vi "Lin_Rohner_lab4A_Stiction torque.vi"() -> ()   [LabVIEW 2019]
uses:
  <vilib>/Analysis/3filter.llb/Filter Passband Type.ctl
  <vilib>/Platform/TimedLoop/XDataNode/timing_clust.ctl
  <vilib>/Platform/TimedLoop/XDataNode/nitl_modes.ctl
  <vilib>/Platform/TimedLoop/XDataNode/wakeup.ctl
  <vilib>/DAQmx/write.llb/DAQmx Write (Analog DBL 1Chan 1Samp).vi
  <vilib>/DAQmx/read.llb/DAQmx Read (Analog DBL 1Chan 1Samp).vi
  <vilib>/DAQmx/create/channels.llb/DAQmx Create Channel (AO-Voltage-Basic).vi
  <vilib>/DAQmx/miscellaneous.llb/DAQmx Fill In Error Info.vi
  <vilib>/DAQmx/create/channels.llb/DAQmx Create Channel (AI-Voltage-Basic).vi
  <vilib>/platform/TimedLoop/XDataNode/XDataNode.xnode
  <vilib>/Platform/TimedLoop/XDataNode/XDNodeRunTimeDep.lvlib
  <vilib>/ptbypt/NI_PtbyPt.lvlib
  <vilib>/Analysis/NI_AALBase.lvlib
panel:
  out "Start Position":dbl
  out "Delta Position":dbl
  in  "Go!":bool
  out "Filtered Position":dbl(graph)
  out "Filtered Position":dbl
  in  "low cutoff freq: Position":dbl=0.125 format="%0.3f"
  out "Motor Voltage":dbl
  out "Motor Current":dbl(graph)
  out "Motor Current":dbl
  out "Motor Control Voltage":dbl(graph)
  in  "Stop!":bool
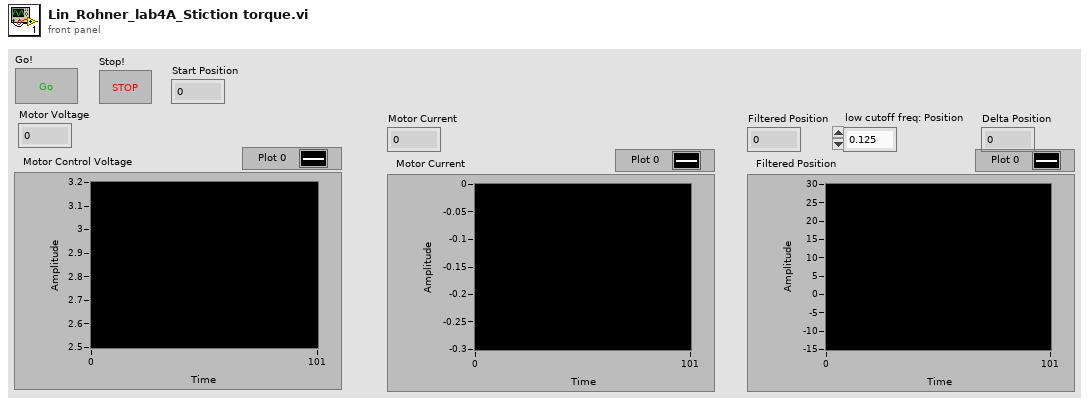
[diagram p1: front panel]
types:
  T1 = typedef "NI_AALBase.lvlib/Filter Passband Type.ctl" = enum32{"Lowpass", "Highpass", "Bandpass", "Bandstop"}
  T2 = typedef "XDNodeRunTimeDep.lvlib/timing_clust.ctl" = cluster{"Expected End [f-1]":u64, "Actual End [f-1]":u64, "Finished Late? [f-1]":bool, "Expected End [i-1]":u64, "Actual End [i-1]":u64, "Finished Late? [i-1]":bool, "Expected Start [i]":u64, "Actual Start [i]":u64, "Expected Start [f]":u64, "Actual Start [f]":u64, "Source Name":string, "Structure Name":string, "Period":i64, "Deadline":i64, "Offset":i64, "Start":i64, "Priority":i32, "Timeout":i32, "Mode":T3, "Wakeup Reason":T4, "Error":errorcluster, "Source Type":string, "Secondary Source Type":string, "Global End Time":u64, "Global Start Time":u64, "Frame Duration":u64, "Iteration Duration":u64, "Assigned CPU":i32, "I/O Scan Engine Mode":u32}
  T3 = typedef "XDNodeRunTimeDep.lvlib/nitl_modes.ctl" = enum32{"No Change", "Process missed periods, maintain original phase", "Discard missed periods, maintain original phase", "Process missed periods, ignore original phase", "Discard missed periods, ignore original phase"}
  T4 = typedef "XDNodeRunTimeDep.lvlib/wakeup.ctl" = enum32{"Normal", "Aborted", "Asynchronous wakeup", "Timing source error", "Timed loop error", "Timeout"}
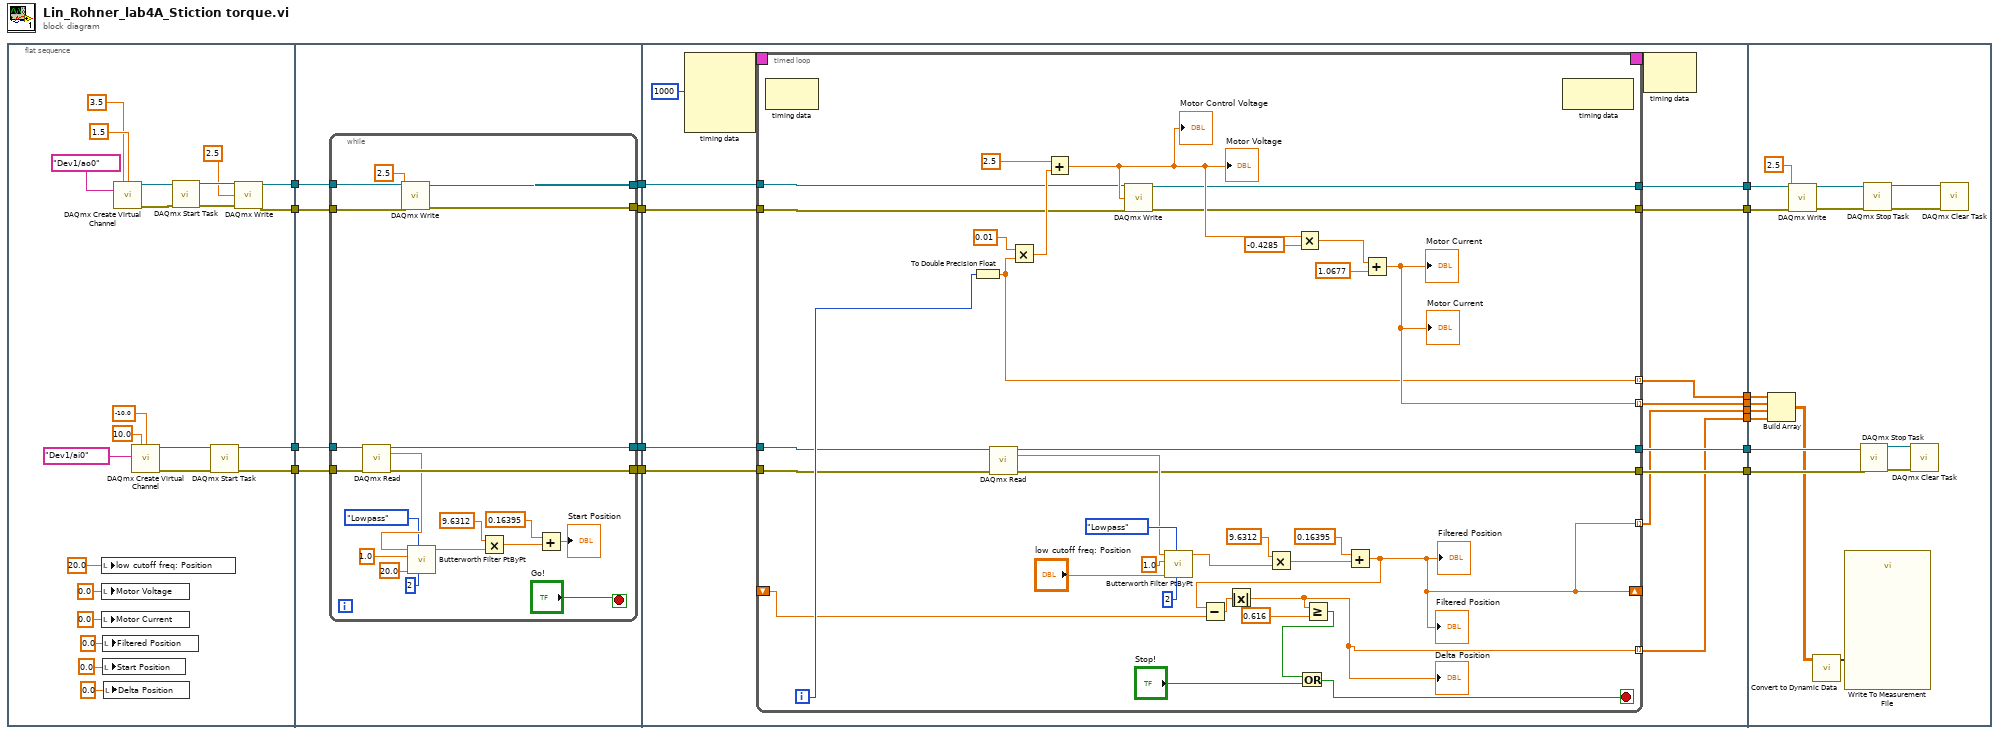
[diagram p0: block diagram]
diagram:
  n1 = flat-sequence {
    tunnel: [w37] -> w11
    tunnel: [w36] -> w9
    tunnel: [w24] -> w7
    tunnel: [w23] -> w5
    tunnel: w11 -> [w47]
    tunnel: [w45] -> w10
    tunnel: w9 -> [w46]
    tunnel: [w44] -> w8
    tunnel: w7 -> [w43]
    tunnel: [w40] -> w6
    tunnel: w5 -> [w42]
    tunnel: [w41] -> w4
    tunnel: w10 -> [w79]
    tunnel: w8 -> [w78]
    tunnel: w6 -> [w77]
    tunnel: w4 -> [w76]
    tunnel: [w75] -> w16
    tunnel: [w74] -> w15
    tunnel: [w73] -> w14
    tunnel: [w72] -> w13
    tunnel: [w71] -> w12
    tunnel: [w70] -> w3
    tunnel: [w69] -> w2
    tunnel: [w68] -> w1
    tunnel: w16 -> [w133]
    tunnel: w15 -> [w132]
    tunnel: w14 -> [w131]
    tunnel: w13 -> [w130]
    tunnel: w12 -> [w128]
    tunnel: w3 -> [w129]
    tunnel: w2 -> [w124]
    tunnel: w1 -> [w125]
    frame #0 {
      n2 = local write "low cutoff freq: Position"(20.0 ("low cutoff freq: Position")) -> ()
      n3 = local write "Motor Voltage"(0.0 ("Motor Voltage")) -> ()
      n4 = local write "Motor Current"(0.0 ("Motor Current")) -> ()
      n5 = local write "Filtered Position"(0.0 ("Filtered Position")) -> ()
      n6 = local write "Start Position"(0.0 ("Start Position")) -> ()
      n7 = local write "Delta Position"(0.0 ("Delta Position")) -> ()
      n8 = call-poly <vilib>:"DAQmx Create Virtual Channel.vi"("maximum value"=3.5, "minimum value"=1.5, "physical channels"=tag "Dev1/ao0") -> ("task out"=w39:refnum<k21>, "error out"=w35:errorcluster)  [unwired: 11 in]
      n9 = call-poly <vilib>:"DAQmx Create Virtual Channel.vi"("maximum value"=10.0, "minimum value"=-10.0, "physical channels"=tag "Dev1/ai0") -> ("task out"=w25:refnum<k21>, "error out"=w26:errorcluster)  [unwired: 11 in]
      n10 = call <vilib>:"DAQmx Start Task.vi"("task/channels in"=w39, "error in"=w35) -> ("task out"=w38:refnum<k21>, "error out"=w34:errorcluster)  [unwired: 12 in]
      n11 = call <vilib>:"DAQmx Start Task.vi"("task/channels in"=w25, "error in"=w26) -> ("task out"=w24:refnum<k21>, "error out"=w23:errorcluster)  [unwired: 12 in]
      n12 = call-poly <vilib>:"DAQmx Write.vi"("task/channels in"=w38, "data"=2.5, "error in"=w34) -> ("task out"=w37:refnum<k21>, "error out"=w36:errorcluster)  [unwired: 10 in, 1 out]
    }
    frame #1 {
      n13 = while {
        tunnel: w47 -> [w67]
        tunnel: w46 -> [w65]
        tunnel: [w66] -> w45
        tunnel: [w64] -> w44
        tunnel: w43 -> [w61]
        tunnel: w42 -> [w58]
        tunnel: [w59] -> w41
        tunnel: [w60] -> w40
        stop <- "Go!" stop-if-true
        n14 = call-poly <vilib>:"DAQmx Read.vi"("task/channels in"=w61, "error in"=w58) -> ("task out"=w60:refnum<k21>, "data"=w57:dbl, "error out"=w59:errorcluster)  [unwired: 11 in]
        n15 = call-poly <vilib>:"DAQmx Write.vi"("task/channels in"=w67, "data"=2.5, "error in"=w65) -> ("task out"=w66:refnum<k21>, "error out"=w64:errorcluster)  [unwired: 10 in, 1 out]
        n16 = call <vilib>:"Butterworth Filter PtByPt.vi"("order"=2, "filter type"=Filter_Passband_Type."Lowpass", "low cutoff freq: fl"=20.0, "sampling freq: fs"=1.0, "x"=w57) -> ("Filtered x"=w49:dbl)  [unwired: 4 in, 1 out]
        n17 = Multiply(x=9.6312, y=w49) -> (x*y=w51:dbl)
        n18 = Add(x=0.16395, y=w51) -> (x+y=→"Start Position":dbl)
      }
    }
    frame #2 {
      n19 = node-c288(i64 1000 ("Period")) -> (w82:T2)  [unwired: 3 in]
      n20 = timed-loop {
        timing: w82 -> [_]
        timing-out: [_] -> w81
        tunnel: w79 -> [w101]
        tunnel: w78 -> [w100]
        tunnel: w77 -> [w97]
        tunnel: w76 -> [w96]
        tunnel: [w99] -> w75
        tunnel: [w98] -> w74
        tunnel: [w95] -> w73
        tunnel: [w94] -> w72
        tunnel: [w89] -> w71 mode=indexing
        shift-right: [w83] -> _
        shift-left: _ -> [w87]
        tunnel: [w85] -> w70 mode=indexing
        tunnel: [w84] -> w69 mode=indexing
        tunnel: [w83] -> w68 mode=indexing
        i -> [w102]
        stop <- w90 stop-if-true
        n21 = node-c288() -> ()  [unwired: 1 in, 1 out]
        n22 = To Double Precision Float(number=w102) -> (double precision float=w85:dbl)
        n23 = call-poly <vilib>:"DAQmx Read.vi"("task/channels in"=w97, "error in"=w96) -> ("task out"=w95:refnum<k21>, "data"=w103:dbl, "error out"=w94:errorcluster)  [unwired: 11 in]
        n24 = Multiply(x=0.01, y=w85) -> (x*y=w116:dbl)
        n25 = Add(x=2.5, y=w116) -> (x+y=w111:dbl)
        "Motor Control Voltage" <- w111
        "Motor Voltage" <- w111
        n26 = call-poly <vilib>:"DAQmx Write.vi"("task/channels in"=w101, "data"=w111, "error in"=w100) -> ("task out"=w99:refnum<k21>, "error out"=w98:errorcluster)  [unwired: 10 in, 1 out]
        n27 = call <vilib>:"Butterworth Filter PtByPt.vi"("order"=2, "filter type"=Filter_Passband_Type."Lowpass", "low cutoff freq: fl"="low cutoff freq: Position", "sampling freq: fs"=1.0, "x"=w103) -> ("Filtered x"=w104:dbl)  [unwired: 4 in, 1 out]
        n28 = Multiply(x=9.6312, y=w104) -> (x*y=w106:dbl)
        n29 = Multiply(x=w111, y=-0.4285) -> (x*y=w113:dbl)
        n30 = Add(x=0.16395, y=w106) -> (x+y=w83:dbl)
        "Filtered Position" <- w83
        "Filtered Position" <- w83
        n31 = Subtract(x=w83, y=w87) -> (x-y=w86:dbl)
        n32 = Absolute Value(x=w86) -> (abs(x)=w84:dbl)
        "Delta Position" <- w84
        n33 = Greater Or Equal?(x=w84, y=0.616) -> (x >= y?=w92:bool)
        n34 = Or(x=w92, y="Stop!") -> (x .or. y?=w90:bool)
        n35 = Add(x=w113, y=1.0677) -> (x+y=w89:dbl)
        "Motor Current" <- w89
        "Motor Current" <- w89
        n36 = node-c288() -> ()  [unwired: 1 in, 1 out]
      }
      n37 = node-c288(w81) -> ()  [unwired: 1 out]
    }
    frame #3 {
      n38 = Build Array(w129, w128, w125, w124) -> (w127:dbl[][])
      n39 = call-poly <vilib>:"DAQmx Write.vi"("task/channels in"=w133, "data"=2.5, "error in"=w132) -> ("task out"=w140:refnum<k21>, "error out"=w137:errorcluster)  [unwired: 10 in, 1 out]
      n40 = call "Convert to Dynamic Data"("2D Array"=w127) -> ("Dynamic Data Type"=w126:dynamicdata)  [unwired: 3 in]
      n41 = call "Write To Measurement File"("Signals"=w126) -> ()  [unwired: 16 in, 3 out]
      n42 = call <vilib>:"DAQmx Stop Task.vi"("task/channels in"=w131, "error in"=w130) -> ("task out"=w134:refnum<k21>, "error out"=w135:errorcluster)  [unwired: 12 in]
      n43 = call <vilib>:"DAQmx Stop Task.vi"("task/channels in"=w140, "error in"=w137) -> ("task out"=w139:refnum<k21>, "error out"=w138:errorcluster)  [unwired: 12 in]
      n44 = call <vilib>:"DAQmx Clear Task.vi"("task in"=w134, "error in"=w135) -> ()  [unwired: 13 in, 1 out]
      n45 = call <vilib>:"DAQmx Clear Task.vi"("task in"=w139, "error in"=w138) -> ()  [unwired: 13 in, 1 out]
    }
  }
